vi "RTS MX100 Read Config.vi"(8 "Error In":errorcluster, 9 "RTS Config Setup":T1, 10 "Config Filenames":string[](array[string]), 11 "Search File Path":path) -> (0 "Error Out":errorcluster, 1 "RTS Config Setup Output":T1, 2 "Config Filenames Output":string[](array[string]), 3 "Search File Path 2":path)   [LabVIEW 2020]
uses:
  Type Definitions/RTS Configuration Setup.ctl
  Type Definitions/RTS Wago Config.ctl
  Type Definitions/RTS APLUS Config.ctl
  Type Definitions/RTS Yokogawa MX Config.ctl
  Type Definitions/RTS Replay Server Control.ctl
  Type Definitions/RTS Server Configuration.ctl
  Type Definitions/RTS Station Settions TCP Comms.ctl
  Type Definitions/RTS Chamber Save Status.ctl
  Type Definitions/RTS Test Pattern.ctl
  <vilib>/Utility/file.llb/Read Delimited Spreadsheet (string).vi
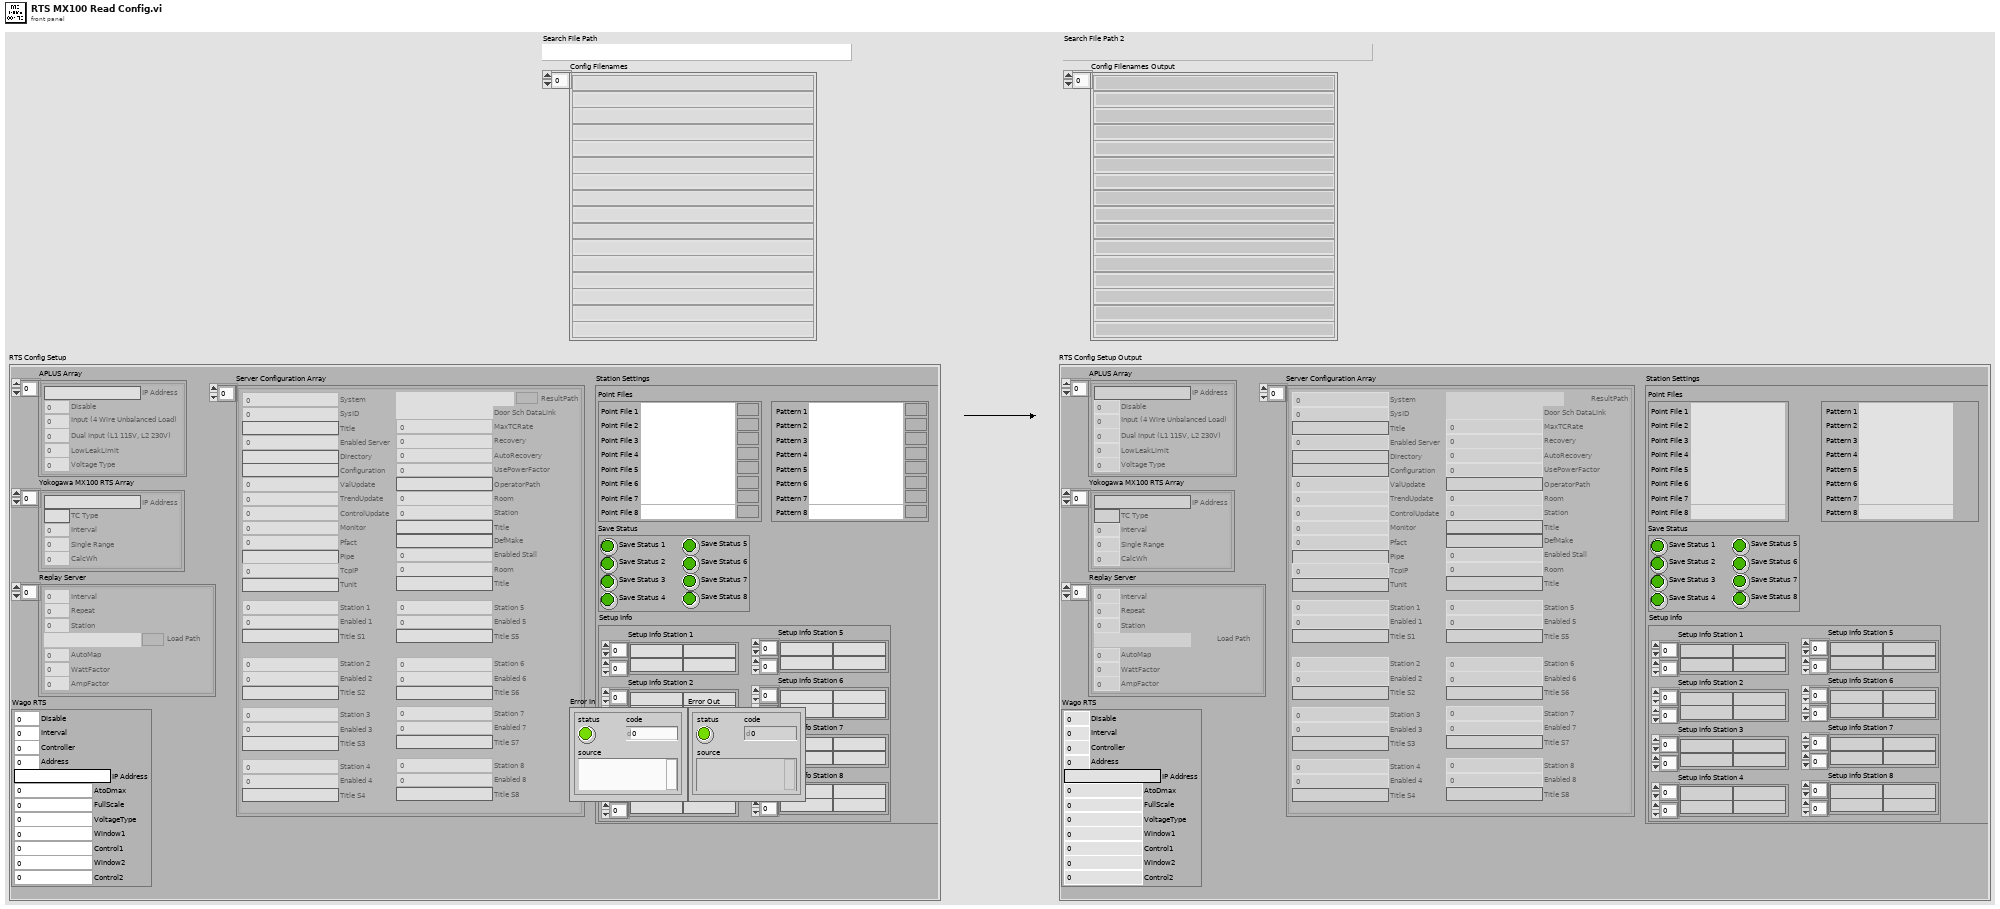
[diagram p1: front panel]
types:
  T1 = typedef "RTS Configuration Setup.ctl" = cluster{"Wago RTS":T2, "APLUS Array":T3[], "Yokogawa MX100 RTS Array":T4[], "Replay Server":T5[], "Server Configuration Array":T6[], "Station Settings":T7}
  T2 = typedef "RTS Wago Config.ctl" = cluster{"Disable":u16, "Interval":u16, "Controller":u16, "Address":u16, "IP Address":string, "AtoDmax":u16, "FullScale":u16, "VoltageType":u16, "Window1":u16, "Control1":u16, "Window2":u16, "Control2":u16}
  T3 = typedef "RTS APLUS Config.ctl" = cluster{"Disable":u16, "IP Address":string, "Input (4 Wire Unbalanced Load)":u16, "Dual Input (L1 115V, L2 230V)":u16, "LowLeakLimit":dbl, "Voltage Type":u16}
  T4 = typedef "RTS Yokogawa MX Config.ctl" = cluster{"IP Address":string, "TC Type":string, "Interval":u16, "Single Range":u16, "CalcWh":u16}
  T5 = typedef "RTS Replay Server Control.ctl" = cluster{"Interval":i16, "Repeat":u16, "Station":u16, "Load Path":path, "AutoMap":u16, "WattFactor":dbl, "AmpFactor":dbl}
  T6 = typedef "RTS Server Configuration.ctl" = cluster{"System":u16, "SysID":u16, "Title":string, "Enabled Server":u16, "Directory":string, "Configuration":string, "ValUpdate":u16, "TrendUpdate":u16, "ControlUpdate":u16, "Monitor":u16, "Pfact":u16, "Pipe":string, "TcpIP":u16, "Tunit":string, "ResultPath":path, "Door Sch DataLink":path, "MaxTCRate":u16, "Recovery":u16, "AutoRecovery":u16, "UsePowerFactor":u16, "OperatorPath":string, "Room":u16, "Station":u16, "Title":string, "DefMake":string, "Enabled Stall":u16, "Room":u16, "Title":string, "Station 1":u16, "Enabled 1":u16, "Station 2":u16, "Enabled 2":u16, "Station 3":u16, "Enabled 3":u16, "Station 4":u16, "Enabled 4":u16, "Station 5":u16, "Enabled 5":u16, "Station 6":u16, "Enabled 6":u16, "Station 7":u16, "Enabled 7":u16, "Station 8":u16, "Enabled 8":u16, "Title S1":string, "Title S2":string, "Title S3":string, "Title S5":string, "Title S6":string, "Title S7":string, "Title S8":string, "Title S4":string}
  T7 = typedef "RTS Station Settions TCP Comms.ctl" = cluster{"Point Files":cluster{"Point File 1":path, "Point File 2":path, "Point File 3":path, "Point File 4":path, "Point File 5":path, "Point File 6":path, "Point File 7":path, "Point File 8":path}, "Save Status":T8, "Setup Info":cluster{"Setup Info Station 1":string[][], "Setup Info Station 2":string[][], "Setup Info Station 3":string[][], "Setup Info Station 4":string[][], "Setup Info Station 5":string[][], "Setup Info Station 6":string[][], "Setup Info Station 7":string[][], "Setup Info Station 8":string[][]}, "Chamber Test Pattern":T9}
  T8 = typedef "RTS Chamber Save Status.ctl" = cluster{"Save Status 1":bool, "Save Status 2":bool, "Save Status 3":bool, "Save Status 4":bool, "Save Status 5":bool, "Save Status 6":bool, "Save Status 7":bool, "Save Status 8":bool}
  T9 = typedef "RTS Test Pattern.ctl" = cluster{" Pattern 1":path, "Pattern 2":path, "Pattern 3":path, "Pattern 4":path, "Pattern 5":path, "Pattern 6":path, "Pattern 7":path, "Pattern 8":path}
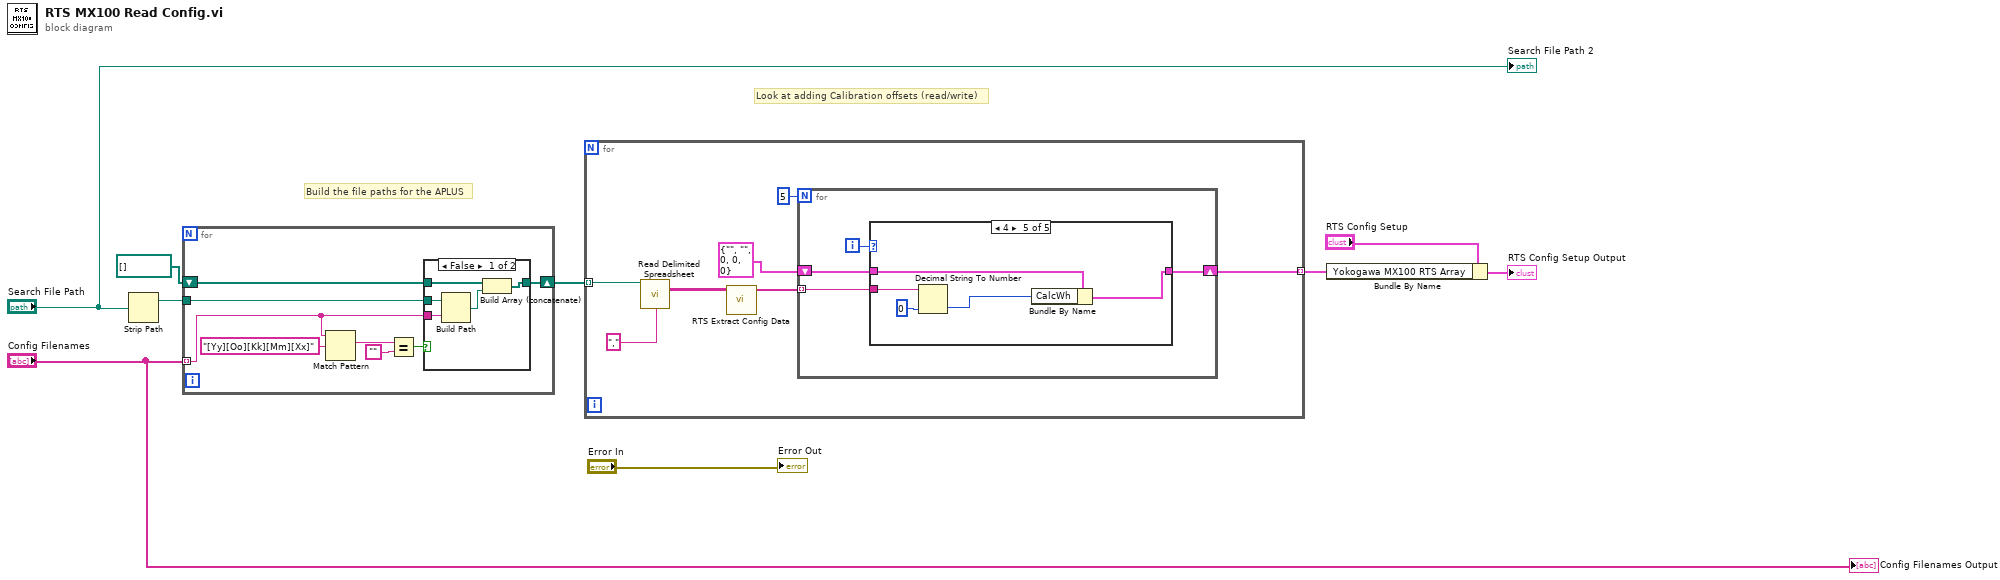
[diagram p0: block diagram]
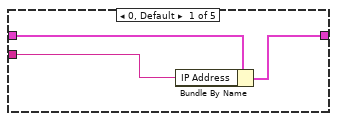
[diagram p2: hidden frame]
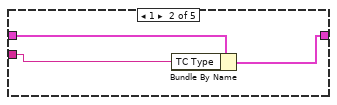
[diagram p3: hidden frame]
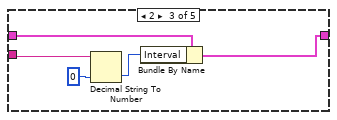
[diagram p4: hidden frame]
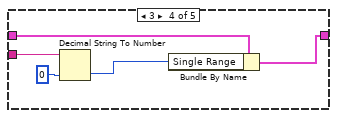
[diagram p5: hidden frame]
diagram:
  # "Look at adding Calibration offsets (read/write)"
  # "Build the file paths for the APLUS"
  n1 = Strip Path(path="Search File Path") -> (stripped path=w6:path)  [unwired: 1 out]
  n2 = for {
    tunnel: "Config Filenames" -> [w10] mode=indexing
    shift-right: [w12] -> w5
    shift-left: path[] [] -> [w13]
    tunnel: w6 -> [w11]
    n3 = Match Pattern(string=w10, regular expression="[Yy][Oo][Kk][Mm][Xx]") -> (match substring=w16:string)  [unwired: 1 in, 3 out]
    n4 = Equal?(x=w16, y="") -> (x = y?=w14:bool)
    n5 = case shown="False" w14 {
      tunnel: w13 -> [w22 w23]
      tunnel: [w21 w23] -> w12
      tunnel: w11 -> [w20 _]
      tunnel: w10 -> [w19 _]
      frame False {
        n6 = Build Path(base path=w20, name or relative path=w19) -> (appended path=w18:path)
        n7 = Build Array (concatenate)(w22, w18) -> (w21:path[])
      }
      frame True {
      }
    }
  }
  n8 = for {
    tunnel: w5 -> [w30] mode=indexing
    tunnel: [w27] -> w3 mode=indexing
    n9 = call-poly <vilib>:"Read Delimited Spreadsheet.vi"("file path (dialog if empty)"=w30, "delimiter (\\t)"="," ("delimiter (\\t)")) -> ("all rows"=w26:string[][])  [unwired: 8 in, 5 out]
    n10 = call "RTS Extract Config Data.vi"("all rows"=w26) -> ("Array"=w24:string[])  [unwired: 9 in, 1 out]
    n11 = for {
      N: 5 -> [_]
      tunnel: w24 -> [w32] mode=indexing
      shift-right: [w33] -> w27
      shift-left: T4 {"IP Address"="", "TC Type"="", "Interval"=0, "Single Range"=0, "CalcWh"=0} ("Yokogawa MX100 RTS") -> [w31]
      i -> [w34]
      n12 = case shown="4" w34 {
        tunnel: w31 -> [w37 w39 w45 w48 w53]
        tunnel: [w36 w40 w44 w47 w52] -> w33
        tunnel: w32 -> [w35 w38 w42 w46 w51]
        frame 0, Default {
          n13 = Bundle By Name(cluster=w37, "IP Address"=w35) -> (w36:T4)
        }
        frame 1 {
          n14 = Bundle By Name(cluster=w39, "TC Type"=w38) -> (w40:T4)
        }
        frame 2 {
          n15 = Decimal String To Number(string=w42, default (0L)=u16 0 ("default (0 I32)")) -> (number=w41:u16)  [unwired: 1 in, 1 out]
          n16 = Bundle By Name(cluster=w45, "Interval"=w41) -> (w44:T4)
        }
        frame 3 {
          n17 = Decimal String To Number(string=w46, default (0L)=u16 0 ("default (0 I32)")) -> (number=w50:u16)  [unwired: 1 in, 1 out]
          n18 = Bundle By Name(cluster=w48, "Single Range"=w50) -> (w47:T4)
        }
        frame 4 {
          n19 = Decimal String To Number(string=w51, default (0L)=u16 0 ("default (0 I32)")) -> (number=w55:u16)  [unwired: 1 in, 1 out]
          n20 = Bundle By Name(cluster=w53, "CalcWh"=w55) -> (w52:T4)
        }
      }
    }
  }
  n21 = Bundle By Name(cluster="RTS Config Setup", "Yokogawa MX100 RTS Array"=w3) -> (→"RTS Config Setup Output":T1)
  "Error Out" <- "Error In"
  "Search File Path 2" <- "Search File Path"
  "Config Filenames Output" <- "Config Filenames"
